vi "TimingChain.vi"() -> ()   [LabVIEW 2012, in "StimulCtrls.lvlib"]
uses:
  StimulCtrls.lvlib
panel:
  in  "Cluster":T1 {"SEQ 5" scale=0.0..20.0 scale format="%#.1g"; "SEQ 4" scale=0.0..20.0 scale format="%#.1g"; "SEQ 3" scale=0.0..20.0 scale format="%#.1g"; "SEQ 2" scale=0.0..20.0 scale format="%#.1g"; "SEQ 1" scale=0.0..20.0 scale format="%#.1g"}
  in  "Max Range 2":dbl
  in  "Max Range":dbl
  in  "Radio Buttons":enum32{"Radio Selection 1", "Radio Selection 2"}(radio)
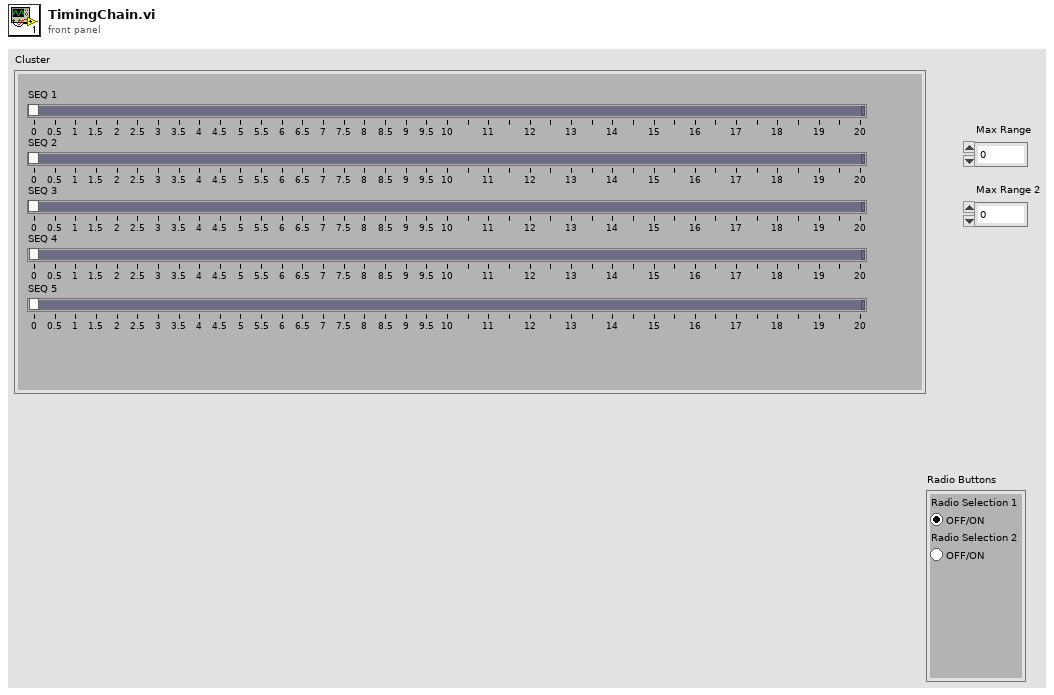
[diagram p1: front panel]
types:
  T1 = cluster{"SEQ 1":cluster{dbl, dbl, dbl}, "SEQ 2":cluster{dbl, dbl, dbl}, "SEQ 3":cluster{dbl, dbl, dbl}, "SEQ 4":cluster{dbl, dbl, dbl}, "SEQ 5":cluster{dbl, dbl, dbl}}
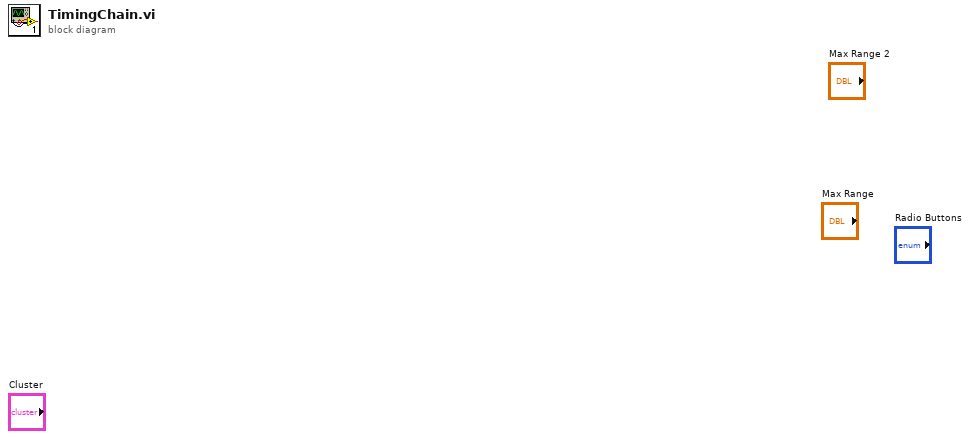
[diagram p0: block diagram]
diagram:
